vi "AlliGator Get 1-Exp Guess Parameters.vi"(9 "IRF":cluster{"t Array":dbl[], "Data Array":dbl[]}, 11 "Decay":cluster{"t Array":dbl[], "Data Array":dbl[]}) -> (0 "Guess Parameters Type":T1, 1 "Guess Parameters Names":T2[](array[typedef]), 3 "Guess Parameters":dbl[](array[numeric]))   [LabVIEW 2021, in "AlliGator Decay Analysis.lvlib" / "AlliGator Decay Fit.lvlib"]
doc: "Determines <B>Guess Parameters</B> for a 1-Exp fit according to the user-specified choices:\n\n* Last valid fitted parameters:\n\nIf the number of available last valid fitted parameters is correct, uses those, otherwise use the estimated parameters.\n\n* User-provided parameters:\n\nIf a parameter is provided by the user, uses it, otherwise uses the estimated parameter.\n\n* User-provided (normalized) parameters:\n\nIf a normalized-parameter (amplitude or baseline) is provided by the user, uses it, otherwise uses the estimated parameter.\n\n* Numerically estimated parameters:\n\nUse the numerically estimated parameters."
uses:
  AlliGator Decay Fit.lvlib
  Fits/IRF(X)PSED/Decay Fit Parameters In List.ctl
  AlliGator Guess Parameters Options.ctl
  AlliGator Settings List.ctl
  Variant/Variant to Data/Variant to [DBL].vi
  <userlib>/_OpenG.lib/array/array.llb/Sort 1D Array (I16)__ogtk.vi
  <userlib>/_OpenG.lib/array/array.llb/Reorder 1D Array2 (DBL)__ogtk.vi
  AlliGator Settings.lvlib
  Variant/Variant to Data/Variant to Data.lvlib
  Fits/Fits.lvlib
  <userlib>/_OpenG.lib/array/array.llb/openg_array.lvlib
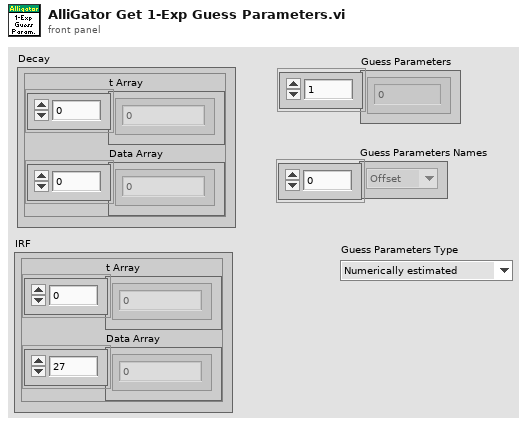
[diagram p1: front panel]
types:
  T1 = typedef "AlliGator Decay Analysis.lvlib/AlliGator Decay Fit.lvlib/AlliGator Guess Parameters Options.ctl" = enum16{"Numerically estimated", "User-provided", "User-provided (normalized)", "Last valid fitted parameters"}
  T2 = typedef "Fits.lvlib/Decay Fit Parameters In List.ctl" = enum16{"Offset", "Baseline", "A_1", "tau_1", "A_2", "tau_2"}
  T3 = typedef "AlliGator Settings.lvlib/AlliGator Settings List.ctl" = enum16{"GUI:Visible Settings Tab", "GUI:Last Run Version", "Source Image:Use Image Histogram for Contrast", "Source Image:Low Count Pixels Rejection Options", "Source Image:High Count Pixels Rejection Options", "Source Image:Use Image Brightness", "Source Image:Blend Overlay with Image Background", "Source Image:Use Fixed ROI Diameter", "Source Image:ROI Diameter", "Source Image:ROI Center Color", "Source Image:Peak Threshold", "Source Image:Intensity Threshold", "Source Image:Image Binning Options", "Source Image:Image Smoothing Options", "Source Image:Image Histogram Active", "Source Image:Invert Binary Mask", "Source Image:Hot Pixel Removal", "Source Image:Overlay Analyzed ROI Center", "Source Image:Auto-Adjust Contrast", "Source Image:Histogram Lower Percentile", "Source Image:Histogram Upper Percentile", "Source Image:Save Source Image", "Source Image:Scale Bar Options", "Source Image:Image Resolution (Pixel Size)", "Source Image:Flatfield Correction", "Source Image:Show Dead Left Columns Correction", "Source Image:Dead Left Columns Correction", "Source Image:Image Pre-Processing Operations Order", "Data Information:Gate Width", "Data Information:Nanotime Gate Separation", "Data Information:Macrotime Gate Separation", "Data Information:Gate Step", "Data Information:# Gates", "Data Information:Gate Image Exposure", "Data Information:Gate Image Integration", "Data Information:Gates to Skip", "Data Information:Gates to Keep", "Data Information:Define Gates to", "Data Information:Channel Name", "Data Information:Available Channel Names", "Data Information:Channel Arithmetic", "Data Information:Background File Subtraction", "Data Information:Background File", "Data Information:Background Scaling Factor", "Data Information:Background Pile-up Correction", "Data Information:Background Pixel Well Capacity", "Data Information:Laser Period", "Data Information:SYNC Period", "Data Information:Pile-up Correction", "Data Information:Pixel Well Capacity", "Data Information:Dataset Scaling Factor", "Fluorescence Decay_Decay Pre-Processing:Reverse Gates", "Fluorescence Decay_Decay Pre-Processing:Verbose Decay Pre-Processing", "Fluorescence Decay_Decay Pre-Processing:Use Decay Pre-Processing", "Fluorescence Decay_Decay Pre-Processing:Background Subtraction", "Fluorescence Decay_Decay Pre-Processing:Background Definition Range", "Fluorescence Decay_Decay Pre-Processing:Baseline Subtraction Method", "Fluorescence Decay_Decay Pre-Processing:Decay Pre-Processing Operations Order", "Fluorescence Decay_Decay Pre-Processing:Smoothing Parameter", "Fluorescence Decay_Decay Pre-Processing:Shift Decay", "Fluorescence Decay_Decay Pre-Processing:Decay Shift Parameters", "Fluorescence Decay_Decay Pre-Processing:Fold Decay", "Fluorescence Decay_Decay Pre-Processing:# Folds", "Fluorescence Decay_Decay Pre-Processing:1-Normalize Decay", "Fluorescence Decay_Decay Pre-Processing:[0-1]-Normalize Decay", "Fluorescence Decay_Decay Pre-Processing:Smoothen Decay", "Fluorescence Decay_Decay Pre-Processing:Extrapolate Decay", "Fluorescence Decay_Decay Pre-Processing:Use Periodicity", "Fluorescence Decay_Decay Pre-Processing:Use Cursors", "Fluorescence Decay_Decay Pre-Processing:Tail Fraction", "Fluorescence Decay_Decay Pre-Processing:Head Fraction", "Fluorescence Decay_Decay Pre-Processing:Additional Points", "Fluorescence Decay_Decay Pre-Processing:Straighten Decay", "Fluorescence Decay_Decay Pre-Processing:Constant Background", "Fluorescence Decay_Decay Pre-Processing:Pixel-Normalize Decay", "Fluorescence Decay_Advanced Analysis:Extract IRF instead of Decay", "Fluorescence Decay_Advanced Analysis:IRF Extraction Options", "Fluorescence Decay_Advanced Analysis:IRF Optimization Options", "Fluorescence Decay_Advanced Analysis:Square Pulse Options", "Fluorescence Decay_Advanced Analysis:IRF Order", "Fluorescence Decay_Advanced Analysis:IRF Time Constants", "Fluorescence Decay_Advanced Analysis:Wavelet Analysis Options", "Fluorescence Decay_Advanced Analysis:Average Lifetime Options", "Fluorescence Decay_Fit Options:Fit Options", "Fluorescence Decay_Fit Options:Use Legacy Fitting Approach", "Fluorescence Decay_Fit Options:Use Data Information Laser Period", "Fluorescence Decay_Fit Parameters:Displayed Fit Parameters", "Fluorescence Decay_Fit Parameters:Fit Parameter Constraints", "Fluorescence Decay_Fit Parameters:Export Tabulated Results", "Fluorescence Decay_Fit Parameters:MLE Baseline Offset Type", "Fluorescence Decay_Fit Parameters:MLE Baseline Offset", "Fluorescence Decay_Fit Parameters:Guess Parameter Names", "Fluorescence Decay_Fit Parameters:Guess Parameter Values", "Fluorescence Decay_Fit Parameters:Guess Parameters Options", "Fluorescence Decay_Styles:Show Last Decay Only", "Fluorescence Decay_Styles:Decay Graph Color Array", "Fluorescence Decay:Decay Graph Active", "Fluorescence Decay Statistics:Min Peak Value", "Fluorescence Decay Statistics:Reject Low Decay Peak Pixels", "Fluorescence Decay Statistics:Reject High Decay Peak Pixels", "Fluorescence Decay Statistics:Max Peak Value", "Time Traces:Use File Timestamp", "Time Traces:Time Step", "Time Traces:Use Intensity Correction File", "Time Traces:Intensity Correction File", "Phasor Plot:Phasor Plot Smoothing Options", "Phasor Plot:Phasor Plot Size", "Phasor Plot:Phasor Plot Graphics Options", "Phasor Plot:Cumulative Phasor Plot", "Phasor Plot:Use Phasor Brightness", "Phasor Plot:Blend Overlay with Phasor Background", "Phasor Plot:Save Phasor Plot", "Phasor Plot:Show References", "Phasor Plot:Phasor Ratio Decay Range", "Phasor Plot:Exponential Fading", "Phasor Plot:Phasor Ratio Reference Colors", "Phasor Plot:Reference Radius", "Phasor Plot:Show Color Map Vertices", "Phasor Plot:Phasor Plot Active", "Phasor Plot:Phasor Ratio Color Map Type", "Phasor Plot:Phasor Ratio Color Map", "Phasor Plot:Phasor Ratio Display Range", "Phasor Plot:Selected Image ROI(s)", "Phasor Plot:All Image ROIs", "Phasor Plot:Selected Phasor Plot ROI(s)", "Phasor Plot:All Phasor Plot ROIs", "Phasor Plot:Phasor Ratio Color-Coded Quantity", "Phasor Plot:Store Phasor Harmonics", "Phasor Plot:Draw Reference Segment", "Phasor Plot:User-Defined Quantity", "Phasor Graph:Phasor Frequency", "Phasor Graph:Phasor Ratio Type", "Phasor Graph:Pixel-level Phasor Computation", "Phasor Graph:Save Phasor Graph", "Phasor Graph:Phasor Graph Active", "Phasor Graph:Phasor SDV Options", "Phasor Calibration:Use Backup Calibration if needed", "Phasor Graph:Define Shortest Lifetime as", "Phasor Calibration:Backup Calibration Type", "Phasor Calibration:Calibration Type", "Phasor Calibration:Calibration Lifetime", "Phasor Calibration:Calibration Map Algorithm", "Single-Exponential Phasor Locus (SEPL):Gate Parameters", "Single-Exponential Phasor Locus (SEPL):User-defined Gate", "Single-Exponential Phasor Locus (SEPL):User-defined IRF", "Single-Exponential Phasor Locus (SEPL):Phasor Parameters", "Single-Exponential Phasor Locus (SEPL):Decay & IRF Parameters", "Single-Exponential Phasor Locus (SEPL):Display Parameters", "Lifetime Analysis:Decay Analysis Parameters", "Lifetime Analysis:Lifetime Map Active", "Plugins:Python Settings", "Miscellaneous:Verbose Mode", "Miscellaneous:Beep after Script", "Miscellaneous:Saved Image File Format", "Miscellaneous:Exported Gate Image Settings", "Miscellaneous:Include Loading in Timing", "Miscellaneous:Verbose Settings Mode", "Miscellaneous:Histogram Options", "Miscellaneous:Beep on Error", "Miscellaneous:# Logical Processors Used", "Miscellaneous:ROI Description Max Characters", "Miscellaneous:Verbose Error Mode", "Miscellaneous:Transparent Mask Color"}
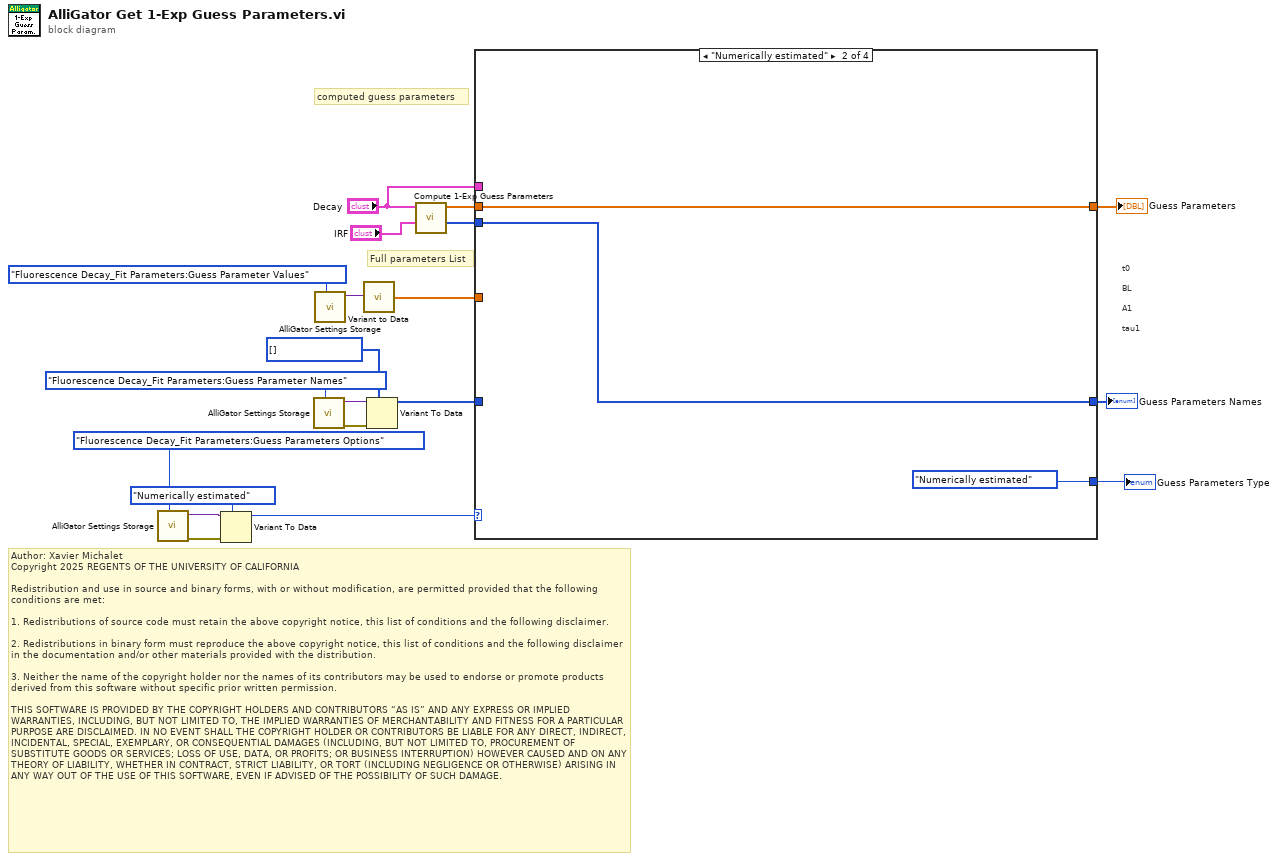
[diagram p0: block diagram]
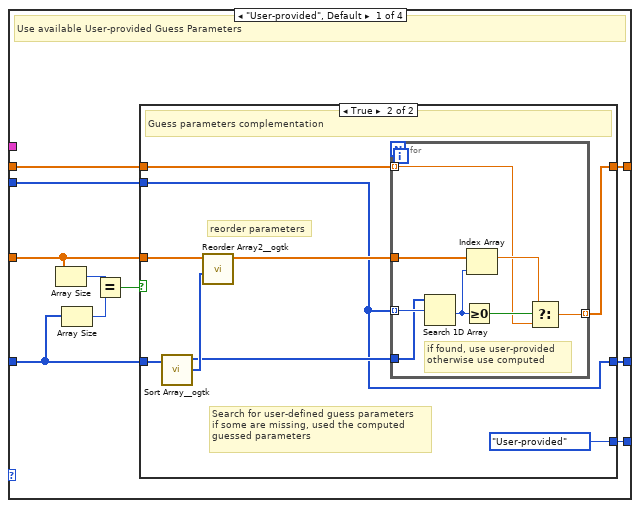
[diagram p2: hidden frame]
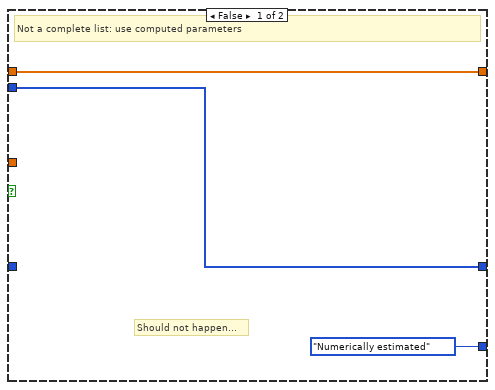
[diagram p3: hidden frame]
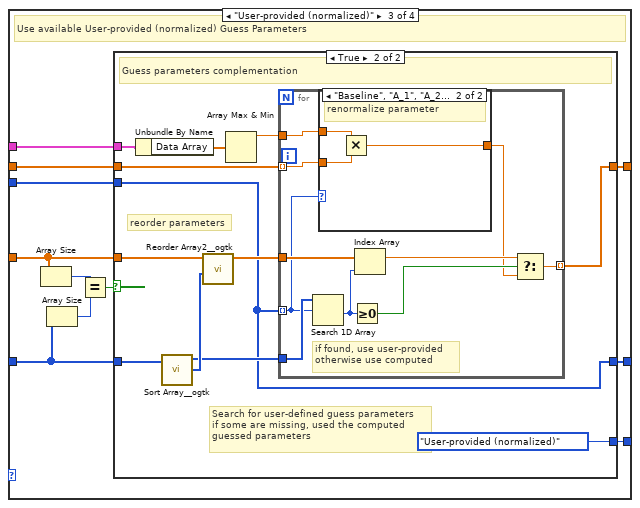
[diagram p4: hidden frame]
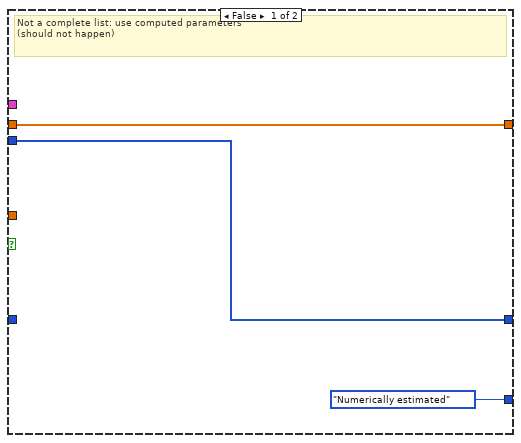
[diagram p5: hidden frame]
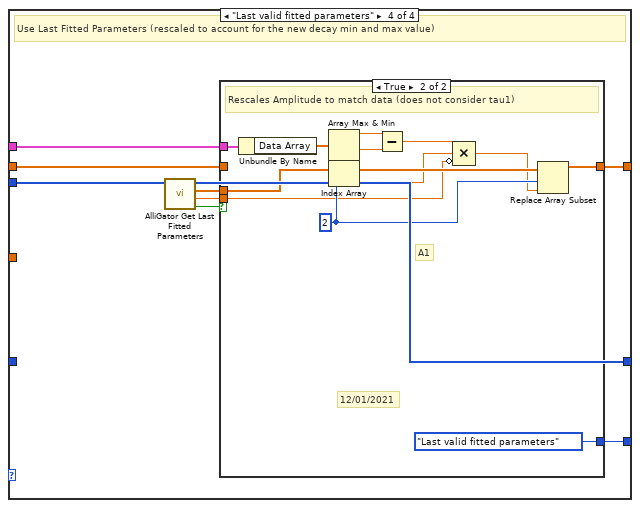
[diagram p7: hidden frame]
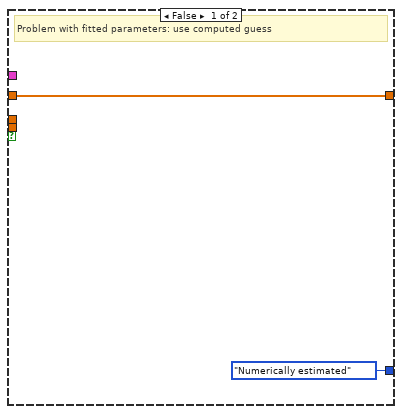
[diagram p8: hidden frame]
diagram:
  w11 = T2[] [] items=["Offset", "Baseline", "A_1", "tau_1", "A_2", "tau_2"] ("Guess Parameters Names")
  # "Author: Xavier Michalet\nCopyright 2025 REGENTS OF THE UNIVERSITY OF CALIFORNIA\n\nRedistribution and use in source and binary forms, with or without modification, are permitted provided that the following conditions are met:\n\n1. Redistributions of source code must retain the above copyright notice, this list of conditions and the following disclaimer.\n\n2. Redistributions in binary form must reproduce the above copyright notice, this list of conditions and the following disclaimer in the documentation and/or other materials provided with the distribution.\n\n3. Neither the name of the copyright holder nor the names of its contributors may be used to endorse or promote products derived from this software without specific prior written permission.\n\nTHIS SOFTWARE IS PROVIDED BY THE COPYRIGHT HOLDERS AND CONTRIBUTORS “AS IS” AND ANY EXPRESS OR IMPLIED WARRANTIES, INCLUDING, BUT NOT LIMITED TO, THE IMPLIED WARRANTIES OF MERCHANTABILITY AND FITNESS FOR A PARTICULAR PURPOSE ARE DISCLAIMED. IN NO EVENT SHALL THE COPYRIGHT HOLDER OR CONTRIBUTORS BE LIABLE FOR ANY DIRECT, INDIRECT, INCIDENTAL, SPECIAL, EXEMPLARY, OR CONSEQUENTIAL DAMAGES (INCLUDING, BUT NOT LIMITED TO, PROCUREMENT OF SUBSTITUTE GOODS OR SERVICES; LOSS OF USE, DATA, OR PROFITS; OR BUSINESS INTERRUPTION) HOWEVER CAUSED AND ON ANY THEORY OF LIABILITY, WHETHER IN CONTRACT, STRICT LIABILITY, OR TORT (INCLUDING NEGLIGENCE OR OTHERWISE) ARISING IN ANY WAY OUT OF THE USE OF THIS SOFTWARE, EVEN IF ADVISED OF THE POSSIBILITY OF SUCH DAMAGE."
  # "Full parameters List"
  # "computed guess parameters"
  # "t0\n\nBL\n\nA1\n\ntau1"
  n1 = call "AlliGator Settings Storage.vi"("AlliGator Settings List"=AlliGator_Settings_List."Fluorescence Decay_Fit Parameters:Guess Parameters Options") -> ("Error Out"=w4:errorcluster, "Variant Data out"=w5:variant)  [unwired: 9 in]
  n2 = Variant To Data(error in=w4, type=AlliGator_Guess_Parameters_Options."Numerically estimated" ("Guess Parameters Options"), Variant=w5) -> (data=w2:T1)  [unwired: 1 out]
  n3 = call "AlliGator Settings Storage.vi"("AlliGator Settings List"=AlliGator_Settings_List."Fluorescence Decay_Fit Parameters:Guess Parameter Names") -> ("Error Out"=w16:errorcluster, "Variant Data out"=w17:variant)  [unwired: 9 in]
  n4 = call "AlliGator Settings Storage.vi"("AlliGator Settings List"=AlliGator_Settings_List."Fluorescence Decay_Fit Parameters:Guess Parameter Values") -> ("Variant Data out"=w20:variant)  [unwired: 9 in, 1 out]
  n5 = call-poly "Variant to Data.vi"("Variant"=w20) -> ("Value"=w14:dbl[])  [unwired: 8 in]
  n6 = Variant To Data(error in=w16, type=w11, Variant=w17) -> (data=w15:T2[])  [unwired: 1 out]
  n7 = call "Compute 1-Exp Guess Parameters.vi"("IRF"="IRF", "Decay"="Decay") -> ("Ordered Guess Parameter Names"=w9:T2[], "Guess Parameters"=w13:dbl[])  [unwired: 8 in]
  n8 = case shown="\"Numerically estimated\"" w2 {
    tunnel: w15 -> [w27 _ w61 _]
    tunnel: w14 -> [w26 _ w60 _]
    tunnel: w13 -> [w25 w53 w59 w102]
    tunnel: [w24 w53 w58 w101] -> w12
    tunnel: [w23 w52 w57 w99] -> w10
    tunnel: w9 -> [w22 w52 w56 w98]
    tunnel: "Decay" -> [_ _ w55 w97]
    tunnel: [w21 AlliGator_Guess_Parameters_Options."Numerically estimated" ("Guess Parameters Options") w54 w94] -> w1
    frame "User-provided", Default {
      # "Use available User-provided Guess Parameters"
      n9 = Array Size(array=w26) -> (size(s)=w28:i32)
      n10 = Array Size(array=w27) -> (size(s)=w30:i32)
      n11 = Equal?(x=w28, y=w30) -> (x = y?=w29:bool)
      n12 = case shown="True" w29 {
        tunnel: w27 -> [_ w42]
        tunnel: w26 -> [_ w41]
        tunnel: w25 -> [w33 w36]
        tunnel: [w33 w37] -> w24
        tunnel: [w32 w35] -> w23
        tunnel: w22 -> [w32 w35]
        tunnel: [AlliGator_Guess_Parameters_Options."Numerically estimated" ("Guess Parameters Options") AlliGator_Guess_Parameters_Options."User-provided" ("Guess Parameters Options")] -> w21
        frame False {
          # "Should not happen..."
          # "Not a complete list: use computed parameters"
        }
        frame True {
          # "reorder parameters"
          # "Search for user-defined guess parameters\nif some are missing, used the computed\nguessed parameters"
          # "Guess parameters complementation"
          n13 = call-poly <userlib>:"Sort Array__ogtk.vi"("Array in"=w42) -> ("Sorted Pointers"=w40:i32[], "Sorted Array out"=w38:i16[])  [unwired: 9 in]
          n14 = call-poly <userlib>:"Reorder Array2__ogtk.vi"("indices"=w40, "array"=w41) -> ("reordered array"=w39:dbl[])  [unwired: 9 in]
          n15 = for {
            tunnel: w39 -> [w47]
            tunnel: w38 -> [w49]
            tunnel: w35 -> [w50] mode=indexing
            tunnel: [w44] -> w37 mode=indexing
            tunnel: w36 -> [w43] mode=indexing
            # "if found, use user-provided\notherwise use computed"
            n16 = Search 1D Array(1D array=w49, element=w50) -> (index of element=w45:i32)  [unwired: 1 in]
            n17 = Greater Or Equal To 0?(x=w45) -> (x >= 0?=w48:bool)
            n18 = Index Array(array=w47, index=w45) -> (element=w46:dbl)
            n19 = Select(t=w46, s=w48, f=w43) -> (s? t:f=w44:dbl)
          }
        }
      }
    }
    frame "Numerically estimated" {
    }
    frame "User-provided (normalized)" {
      # "Use available User-provided (normalized) Guess Parameters"
      n20 = Array Size(array=w60) -> (size(s)=w62:i32)
      n21 = Array Size(array=w61) -> (size(s)=w64:i32)
      n22 = Equal?(x=w62, y=w64) -> (x = y?=w63:bool)
      n23 = case shown="True" w63 {
        tunnel: w61 -> [_ w79]
        tunnel: w60 -> [_ w78]
        tunnel: w59 -> [w67 w73]
        tunnel: [w67 w74] -> w58
        tunnel: [w66 w72] -> w57
        tunnel: w56 -> [w66 w72]
        tunnel: w55 -> [_ w71]
        tunnel: [AlliGator_Guess_Parameters_Options."Numerically estimated" ("Guess Parameters Options") AlliGator_Guess_Parameters_Options."User-provided (normalized)" ("Guess Parameters Options")] -> w54
        frame False {
          # "Not a complete list: use computed parameters\n(should not happen)"
        }
        frame True {
          # "reorder parameters"
          # "Search for user-defined guess parameters\nif some are missing, used the computed\nguessed parameters"
          # "Guess parameters complementation"
          n24 = Unbundle By Name(w71) -> ("Data Array"=w70:dbl[])
          n25 = call-poly <userlib>:"Sort Array__ogtk.vi"("Array in"=w79) -> ("Sorted Pointers"=w77:i32[], "Sorted Array out"=w75:i16[])  [unwired: 9 in]
          n26 = call-poly <userlib>:"Reorder Array2__ogtk.vi"("indices"=w77, "array"=w78) -> ("reordered array"=w76:dbl[])  [unwired: 9 in]
          n27 = Array Max & Min(array=w70) -> (max value=w69:dbl)  [unwired: 3 out]
          n28 = for {
            tunnel: w76 -> [w87]
            tunnel: w75 -> [w89]
            tunnel: w72 -> [w83] mode=indexing
            tunnel: [w84] -> w74 mode=indexing
            tunnel: w73 -> [w81] mode=indexing
            tunnel: w69 -> [w82]
            # "if found, use user-provided\notherwise use computed"
            n29 = Search 1D Array(1D array=w89, element=w83) -> (index of element=w85:i32)  [unwired: 1 in]
            n30 = case shown="\"Baseline\", \"A_1\", \"A_2\"" w83 {
              tunnel: w82 -> [_ w93]
              tunnel: w81 -> [w90 w92]
              tunnel: [w90 w91] -> w80
              frame "Offset", Default {
              }
              frame "Baseline", "A_1", "A_2" {
                # "renormalize parameter"
                n31 = Multiply(x=w93, y=w92) -> (x*y=w91:dbl)
              }
            }
            n32 = Greater Or Equal To 0?(x=w85) -> (x >= 0?=w88:bool)
            n33 = Index Array(array=w87, index=w85) -> (element=w86:dbl)
            n34 = Select(t=w86, s=w88, f=w80) -> (s? t:f=w84:dbl)
          }
        }
      }
    }
    frame "Last valid fitted parameters" {
      # "Use Last Fitted Parameters (rescaled to account for the new decay min and max value)"
      n35 = call "AlliGator Get Last Fitted Parameters.vi"("Guess Parameters Names"=w98) -> ("Last Fitted Parameters OK"=w95:bool, "Last Decay Max - Min"=w96:dbl, "Last Fitted Parameters"=w100:dbl[], "Guess Parameters Names (dup)"=w99:T2[])  [unwired: 7 in]
      n36 = case shown="True" w95 {
        tunnel: w102 -> [w104 _]
        tunnel: [w104 w112] -> w101
        tunnel: w100 -> [_ w109]
        tunnel: w97 -> [_ w116]
        tunnel: w96 -> [_ w107]
        tunnel: [AlliGator_Guess_Parameters_Options."Numerically estimated" ("Guess Parameters Options") AlliGator_Guess_Parameters_Options."Last valid fitted parameters" ("Guess Parameters Options")] -> w94
        frame False {
          # "Problem with fitted parameters: use computed guess"
        }
        frame True {
          w110 = 2 ("index")
          # "A1"
          # "12/01/2021"
          # "Rescales Amplitude to match data (does not consider tau1)"
          n37 = Unbundle By Name(w116) -> ("Data Array"=w115:dbl[])
          n38 = Array Max & Min(array=w115) -> (max value=w114:dbl, min value=w113:dbl)  [unwired: 2 out]
          n39 = Index Array(array=w109, index=w110) -> (element=w108:dbl)
          n40 = Subtract(x=w114, y=w113) -> (x-y=w111:dbl)
          n41 = Compound Arithmetic op=MULTIPLY(w111, w108, invert w107) -> (w106:dbl)
          n42 = Replace Array Subset(array=w109, new element=w106, index=w110) -> (w112:dbl[])
        }
      }
    }
  }
  "Guess Parameters" <- w12
  "Guess Parameters Names" <- w10
  "Guess Parameters Type" <- w1
